vi "Write ErrorMessage.vi"(8 "error (to be sent)":errorcluster, 10 "Label":string) -> (0 "error out":errorcluster, 3 "Message":refnum<class "ErrorMessage.lvclass">)   [LabVIEW 2011, in "Messenging.lvlib" / "ErrorMessage.lvclass"]
uses:
  ErrorMessage.lvclass
  ErrorMessage.lvclass/ErrorMessage.ctl
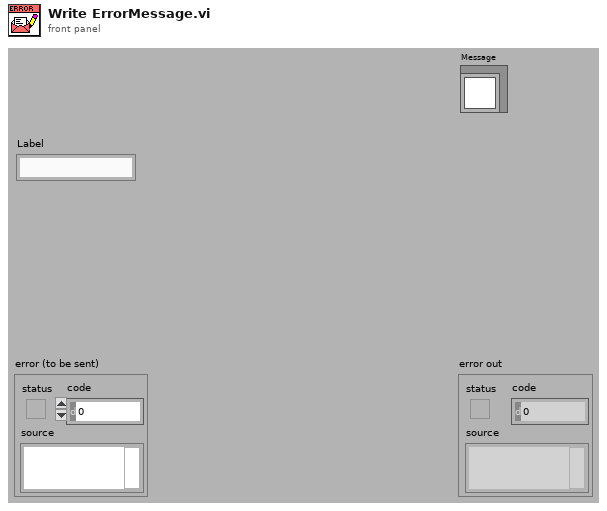
[diagram p1: front panel]
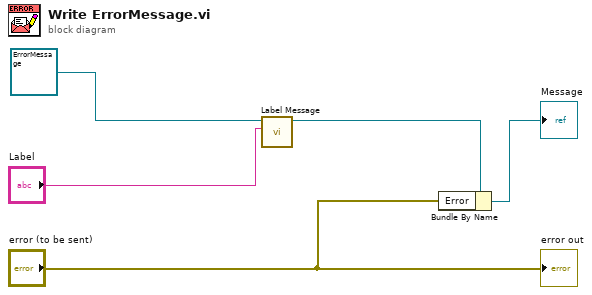
[diagram p0: block diagram]
diagram:
  n1 = call-dynamic "Label Message.vi"("Label"="Label", "Message"=refnum<class "ErrorMessage.lvclass"> refnum ("VarMessage.lvclass")) -> ("Message"=w1:refnum<class "ErrorMessage.lvclass">)  [unwired: 1 in, 8 out]
  n2 = Bundle By Name(cluster=w1, "Error"="error (to be sent)") -> (→"Message":refnum<class "ErrorMessage.lvclass">)
  "error out" <- "error (to be sent)"
